vi "Master RT Target.vi"() -> ()   [LabVIEW 2011]
uses:
  <vilib>/LabVIEW Targets/FPGA/cRIO/cRIO-9505/controls.llb/_nicrio_cRIO-9505_DriveStatus.ctl
  <vilib>/FPGAPlugInAG/cRIO-9074/niLvFpga_Open_cRIO-9074.vi
  <vilib>/Utility/error.llb/Error Cluster From Error Code.vi
  <vilib>/rvi/errors/niLvFpgaAdjustHostInterfaceError.vi
  <vilib>/FPGAPlugInAG/cRIO-9074/niLvFpga_Close_cRIO-9074.vi
  <vilib>/rvi/interface/nirviOpenFPGA/nirviOpenFPGA.xnode
  FPGA/FPGA Bitfiles/MasterInterface.lvbitx
  <vilib>/rvi/interface/nirviReadWriteControl/nirviReadWriteControl.xnode
  <vilib>/rvi/interface/nirviCloseFPGA/nirviCloseFPGA.xnode
  NiFpgaLv.dll
panel:
  in  "Current PID Gains":T1={"Proportional Gain"=20, "Integral Gain"=10, "Derivative Gain"=0}
  in  "Current Limit (A)":dbl min=0.0 max=0.9 step=0.1
  out "Control Status":errorcluster
  in  "Control Rate (ms)":u32=1
  in  "Current Loop Rate (usec)":u32=50
  in  "Stop":bool
  in  "Read Port":u16=9090
  in  "UDP Rate (ms)":u32=1
  in  "Slave IP":string="192.168.10.4"
  out "UDP Status":errorcluster
  in  "Write Port":u16=9595
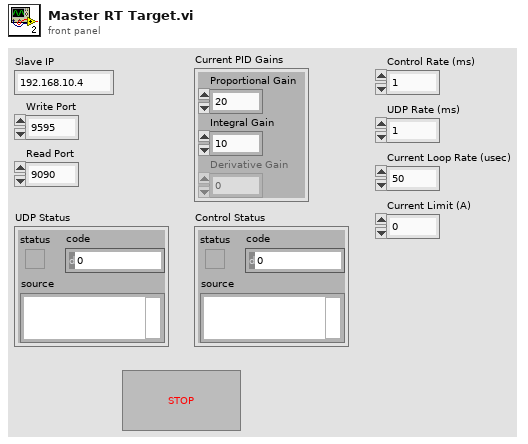
[diagram p1: front panel]
types:
  T1 = cluster{"Proportional Gain":i16, "Integral Gain":i16, "Derivative Gain":i16}
  T2 = typedef "_nicrio_cRIO-9505_DriveStatus.ctl" = enum8{"Enabled", "Disabled", "Disabled by Drive Fault", "Disabled by Temp. Fault", "Disabled by E-Stop", "Unknown"}
  T3 = enum16{"big-endian, network order", "native, host order", "little-endian"}
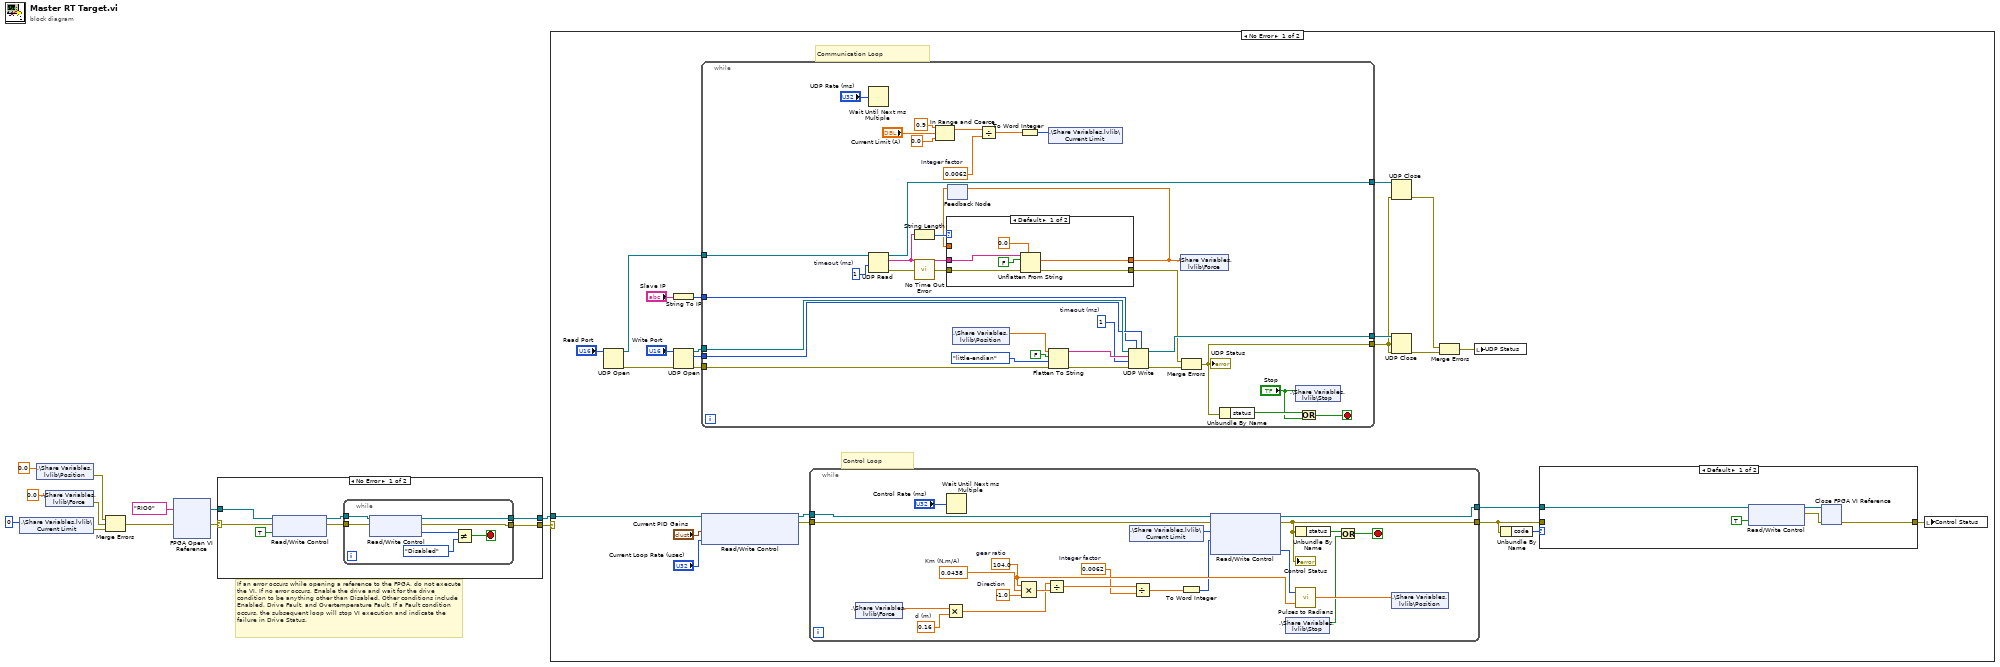
[diagram p0: block diagram]
diagram:
  # "If an error occurs while opening a reference to the FPGA, do not execute the VI. If no error occurs, Enable the drive and wait for the drive condition to be anything other than Disabled. Other conditions include Enabled, Drive Fault, and Overtemperature Fault. If a Fault condition occurs, the subsequent loop will stop VI execution and indicate the failure in Drive Status."
  n1 = shared-variable ".\\Share Variables.lvlib\\Current Limit"(i16 0 ("Current Limit")) -> (error out=w2:errorcluster)  [unwired: 1 in]
  n2 = shared-variable ".\\Share Variables.lvlib\\Position"(0.0 ("Position")) -> (error out=w7:errorcluster)  [unwired: 1 in]
  n3 = shared-variable ".\\Share Variables.lvlib\\Force"(0.0 ("Force")) -> (error out=w6:errorcluster)  [unwired: 1 in]
  n4 = Merge Errors(w7, w6, w2) -> (w5:errorcluster)
  n5 = xnode "FPGA Open VI Reference"("error in"=w5, "resource name"=tag "RIO0") -> ("FPGA VI Reference Out"=w12:refnum<k20>, "error out"=w11:errorcluster)
  n6 = case shown="No Error" w11 {
    selector: w11 -> [w14 w27]
    tunnel: w12 -> [w15 w28]
    tunnel: [w19 w28] -> w3
    tunnel: [w16 w27] -> w4
    frame No Error {
      n7 = xnode "Read/Write Control"("FPGA VI Reference In"=w15, "error in"=w14, "Enable Drive"=TRUE) -> ("FPGA VI Reference Out"=w18:refnum<k20>, "error out"=w17:errorcluster)
      n8 = while {
        tunnel: [w26] -> w19
        tunnel: w18 -> [w23]
        tunnel: w17 -> [w22]
        tunnel: [w24] -> w16
        stop <- w20 stop-if-true
        n9 = xnode "Read/Write Control"("FPGA VI Reference In"=w23, "error in"=w22) -> ("FPGA VI Reference Out"=w26:refnum<k20>, "error out"=w24:errorcluster, "Drive Status"=w21:T2)
        n10 = Not Equal?(x=w21, y=_nicrio_cRIO-9505_DriveStatus."Disabled") -> (x != y?=w20:bool)
      }
    }
    frame Error {
      # "Error occurred. Do not run."
    }
  }
  n11 = case shown="No Error" w4 {
    tunnel: w3 -> [w40 _]
    frame No Error {
      # "Control Loop"
      # "Communication Loop"
      n12 = UDP Open(11:"Read Port") -> (port=w45:refnum<k16>, 0:w44:errorcluster)  [unwired: 1 in, 4 out]
      n13 = String To IP(1:"Slave IP") -> (0:w50:u32)
      n14 = UDP Open(8:w44, 11:"Write Port") -> (port=w49:refnum<k16>, 0:w43:errorcluster, 2:w48:u16)  [unwired: 3 out]
      n15 = while {
        tunnel: [w110] -> w47
        tunnel: w49 -> [w109]
        tunnel: w48 -> [w108]
        tunnel: w50 -> [w104]
        tunnel: w45 -> [w101]
        tunnel: [w97] -> w41
        tunnel: w43 -> [w99]
        tunnel: [w96] -> w42
        stop <- w103 stop-if-true
        w87 = 0.0062  # Integer factor
        w89 = 1  # timeout (ms)
        w112 = 1  # timeout (ms)
        n16 = Wait Until Next ms Multiple(millisecond multiple="UDP Rate (ms)") -> ()  [unwired: 1 out]
        n17 = UDP Read(connection ID=w101, timeout ms (25000)=w89) -> (data out=w95:string, error out=w102:errorcluster, 3:w96:refnum<k16>)  [unwired: 2 in, 2 out]
        n18 = String Length(string=w95) -> (length=w100:i32)
        n19 = call <vilib>:"No Time Out Error.vi"("error in (no error)"=w102) -> ("error out"=w94:errorcluster)  [unwired: 14 out]
        n20 = In Range and Coerce(upper limit=0.9 ("element"), x="Current Limit (A)", lower limit=0.0 ("element")) -> (coerced(x)=w81:dbl)  [unwired: 1 out]
        n21 = feedback #1() -> (w91:dbl)  [unwired: 1 in]
        n22 = case shown="Default" w100 {
          tunnel: w95 -> [w118 _]
          tunnel: w94 -> [w117 w122]
          tunnel: [w116 w122] -> w93
          tunnel: [w115 w121] -> w92
          tunnel: w91 -> [_ w121]
          frame Default {
            n23 = Unflatten From String(type=0.0, binary string=w118, data includes array or string size? (T)=FALSE, error in (no error)=w117) -> (value=w115:dbl, error out=w116:errorcluster)  [unwired: 2 out]
          }
          frame 0 {
          }
        }
        n24 = feedback-in #1(w92) -> ()
        n25 = shared-variable ".\\Share Variables.lvlib\\Position"() -> (w90:dbl)  [unwired: 1 in, 1 out]
        n26 = Divide(x=w81, y=w87) -> (x/y=w86:dbl)
        n27 = To Word Integer(number=w86) -> (16bit integer=w85:i16)
        n28 = shared-variable ".\\Share Variables.lvlib\\Current Limit"(w85) -> ()  [unwired: 1 in, 1 out]
        n29 = Flatten To String(anything=w90, prepend array or string size? (T)=FALSE, byte order (0:big-endian, network order)=T3."little-endian" ("Byte order"), error in (no error)=w99) -> (data string=w113:string, error out=w111:errorcluster)  [unwired: 1 out]
        n30 = UDP Write(address=w104, port or service name=w108, connection ID=w109, data in=w113, 8:w111, 9:w112) -> (error out=w98:errorcluster, 3:w110:refnum<k16>)
        n31 = shared-variable ".\\Share Variables.lvlib\\Force"(w92) -> ()  [unwired: 1 in, 1 out]
        n32 = Merge Errors(w93, w98) -> (w97:errorcluster)
        "UDP Status" <- w97
        n33 = Unbundle By Name(w97) -> ("status"=w107:bool)
        n34 = shared-variable ".\\Share Variables.lvlib\\Stop"("Stop") -> ()  [unwired: 1 in, 1 out]
        n35 = Or(x=w107, y="Stop") -> (x .or. y?=w103:bool)
      }
      n36 = xnode "Read/Write Control"("FPGA VI Reference In"=w40, "Current PI Gains"="Current PID Gains", "Current Loop Rate (usec)"="Current Loop Rate (usec)") -> ("FPGA VI Reference Out"=w39:refnum<k20>, "error out"=w38:errorcluster)  [unwired: 1 in]
      n37 = while {
        tunnel: w39 -> [w80]
        tunnel: w38 -> [w77]
        tunnel: [w64] -> w35
        tunnel: [w59] -> w34
        stop <- w60 stop-if-true
        w66 = 0.16  # d (m)
        w68 = 0.0438  # Km (N.m/A)
        w70 = -1.0  # Direction
        w72 = 0.0062  # Integer factor
        w74 = 104.0  # gear ratio
        n38 = shared-variable ".\\Share Variables.lvlib\\Force"() -> (w67:dbl)  [unwired: 1 in, 1 out]
        n39 = Multiply(x=w67, y=w66) -> (x*y=w65:dbl)
        n40 = Wait Until Next ms Multiple(millisecond multiple="Control Rate (ms)") -> ()  [unwired: 1 out]
        n41 = Compound Arithmetic op=MULTIPLY(w74, w68, w70) -> (w75:dbl)
        n42 = Divide(x=w65, y=w75) -> (x/y=w73:dbl)
        n43 = shared-variable ".\\Share Variables.lvlib\\Current Limit"() -> (w76:i16)  [unwired: 1 in, 1 out]
        n44 = Divide(x=w73, y=w72) -> (x/y=w71:dbl)
        n45 = To Word Integer(number=w71) -> (16bit integer=w69:i16)
        n46 = xnode "Read/Write Control"("FPGA VI Reference In"=w80, "error in"=w77, "Current Limit"=w76, "Current Setpoint"=w69) -> ("FPGA VI Reference Out"=w64:refnum<k20>, "error out"=w59:errorcluster, "Encoder Position"=w79:i32)
        "Control Status" <- w59
        n47 = shared-variable ".\\Share Variables.lvlib\\Stop"() -> (w62:bool)  [unwired: 1 in, 1 out]
        n48 = Unbundle By Name(w59) -> ("status"=w61:bool)
        n49 = call "Pulses to Radians.vi"("gear ratio"=w74, "encoder pulses"=w79) -> ("angle (rad)"=w78:dbl)
        n50 = Or(x=w61, y=w62) -> (x .or. y?=w60:bool)
        n51 = shared-variable ".\\Share Variables.lvlib\\Position"(w78) -> ()  [unwired: 1 in, 1 out]
      }
      n52 = UDP Close(connection ID=w42, 8:w41) -> (error out=w32:errorcluster)  [unwired: 1 out]
      n53 = UDP Close(connection ID=w47, 8:w41) -> (error out=w31:errorcluster)  [unwired: 1 out]
      n54 = Merge Errors(w32, w31) -> (w30:errorcluster)
      n55 = local write "UDP Status"(w30) -> ()
      n56 = Unbundle By Name(w34) -> ("code"=w36:i32)
      n57 = case shown="Default" w36 {
        tunnel: [w55 w58] -> w33
        tunnel: w35 -> [w54 _]
        tunnel: w34 -> [_ w58]
        frame Default {
          n58 = xnode "Read/Write Control"("FPGA VI Reference In"=w54, "Disable Drive"=TRUE ("Disable Motors")) -> ("FPGA VI Reference Out"=w57:refnum<k20>, "error out"=w56:errorcluster)  [unwired: 1 in]
          n59 = xnode "Close FPGA VI Reference"("FPGA VI Reference In"=w57, "error in"=w56) -> ("error out"=w55:errorcluster)
        }
        frame -65536 {
          # "Unable to communicate with the module. Reinsert the module and check connections.\nIf the chassis is in FPGA Interface programming mode, make sure you have opened an \nFPGA reference to a bitfile or FPGA VI with Scan Interface support for the module you are \ntrying to access using the Scan Interface."
        }
      }
      n60 = local write "Control Status"(w33) -> ()
    }
    frame Error {
    }
  }
